vi "Iterpolate to X.vi"(4 "XY Graph Ref":refnum<vi>, 6 "X column name":string, 7 "group name":string, 8 "error in (no error)":errorcluster, 9 "Settings":string, 10 "Data file path":path, 11 "signal(s) in":waveform(dbl)[](array[waveform])) -> (0 "error out":errorcluster, 1 "Settings out":string, 3 "Signals out":waveform(dbl)[](array[waveform]), 5 "X waveform out":waveform(dbl))   [LabVIEW 2015]
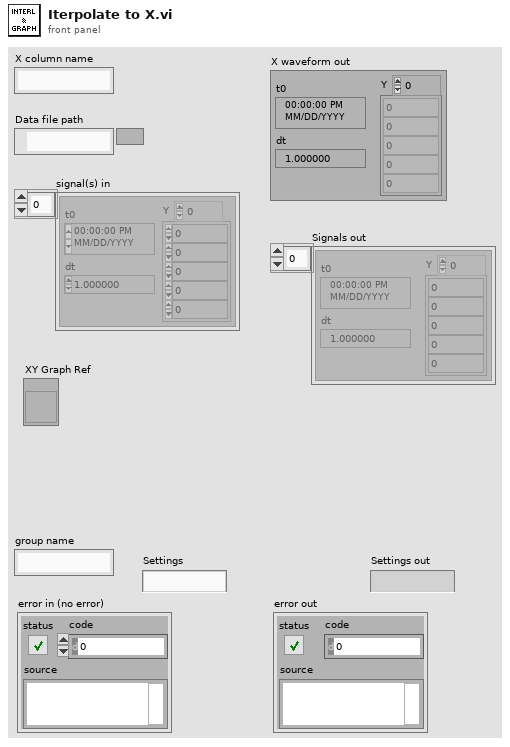
[diagram p1: front panel]
types:
  T1 = enum16{"open", "open or create", "create or replace", "create", "open (read-only)"}
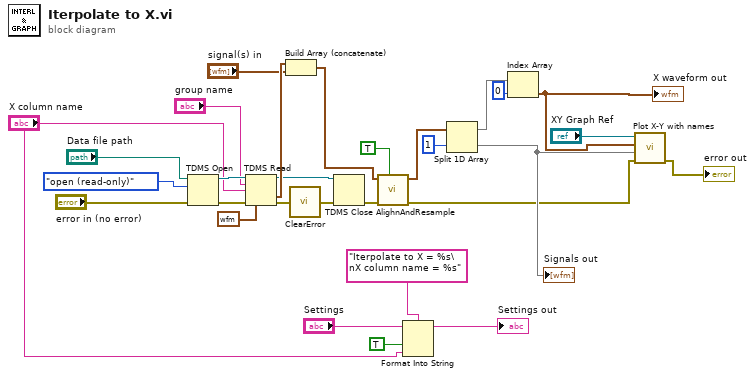
[diagram p0: block diagram]
diagram:
  n1 = TDMS Open(8:"error in (no error)", 10:T1."open (read-only)" ("operation (0:open)"), 11:"Data file path") -> (0:w23:errorcluster, 3:w22:refnum<k34>)  [unwired: 4 in]
  n2 = TDMS Read(0:w22, 5:"group name", 7:"X column name", 11:w23, 12:waveform(sgl) {"t0"=timestamp(0 s since 1904-01-01), "dt"=1.0, "Y"=[]} ("data type")) -> (4:w12:refnum<k34>, 10:w27:waveform(sgl), 15:w18:errorcluster)  [unwired: 3 in, 3 out]
  n3 = Build Array (concatenate)(w27, "signal(s) in") -> (w20:waveform(dbl)[])
  n4 = call <vilib>:"ClearError.vi"("error in (no error)"=w18) -> ("error out"=w28:errorcluster)
  n5 = TDMS Close(8:w28, 11:w12) -> (0:w29:errorcluster)  [unwired: 1 out]
  n6 = call "AlighnAndResample.vi"("Resample to longest dt (F:Resample to shortest dt)"=TRUE ("Resample to longest dt (F:Resample to X dt)"), "error in (no error)"=w29, "waveforms in"=w20) -> ("error out"=w2:errorcluster, "waveforms out"=w21:waveform(dbl)[])  [unwired: 1 in, 6 out]
  n7 = Format Into String(format string="Iterpolate to X = %s\nX column name = %s", initial string="Settings", TRUE, "X column name") -> (resulting string=→"Settings out":string)  [unwired: 1 in, 1 out]
  n8 = Split 1D Array(array=w21, index=1) -> (first subarray=w16:waveform(dbl)[], second subarray=w4:waveform(dbl)[])
  "Signals out" <- w4
  n9 = Index Array(array=w16, index=0) -> (element=w3:waveform(dbl))
  "X waveform out" <- w3
  n10 = call "Plot X-Y with names.vi"("Error In"=w2, "Y columns"=w4, "X column"=w3, "XY Graph Ref"="XY Graph Ref") -> ("Error Out"=→"error out":errorcluster)  [unwired: 6 in, 1 out]
